vi "Subtract - CM,CM.vi"(1 "Complex Matrix B":T1, 2 "Complex Matrix A":T1) -> (0 "A - B":T1)   [LabVIEW 2010, in "NI_Matrix.lvlib"]
doc: "Computes the difference of the inputs."
uses:
  NI_Matrix.lvlib
  ComplexMatrix.ctl
  Matrix To Array - CM.vi
  Array To Matrix - CA2.vi
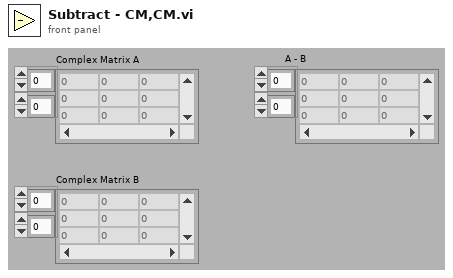
[diagram p1: front panel]
types:
  T1 = typedef "NI_Matrix.lvlib/ComplexMatrix.ctl" = cdb[][]
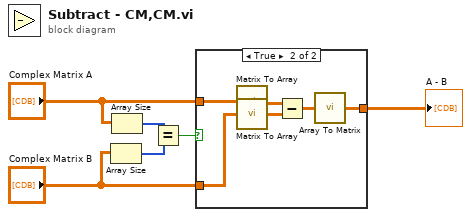
[diagram p0: block diagram]
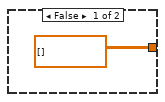
[diagram p2: hidden frame]
diagram:
  n1 = Array Size(array="Complex Matrix B") -> (size(s)=w5:i32[])
  n2 = Array Size(array="Complex Matrix A") -> (size(s)=w6:i32[])
  n3 = Equal?(x=w6, y=w5) -> (x = y?=w4:bool)
  n4 = case shown="True" w4 {
    tunnel: "Complex Matrix A" -> [_ w11]
    tunnel: "Complex Matrix B" -> [_ w10]
    tunnel: [T1 [] ("A - B") w8] -> w1
    frame False {
    }
    frame True {
      n5 = call-poly "Matrix To Array.vi"("Complex Matrix"=w11) -> ("Complex 2D Array"=w12:cdb[][])
      n6 = call-poly "Matrix To Array.vi"("Complex Matrix"=w10) -> ("Complex 2D Array"=w13:cdb[][])
      n7 = Subtract(x=w12, y=w13) -> (x-y=w9:cdb[][])
      n8 = call-poly "Array To Matrix.vi"("Complex 2D Array"=w9) -> ("Complex Matrix"=w8:T1)
    }
  }
  "A - B" <- w1
